vi "Flowmeter2.vi"() -> ()   [LabVIEW 2018]
uses:
  <vilib>/measure/NI_MABase.lvlib
panel:
  out "Waveform Graph 5":dynamicdata(graph)
  out "Waveform Graph 4":waveform(dbl)(graph)
  out "Waveform Graph 3":waveform(dbl)(graph)
  out "Waveform Graph 2":waveform(dbl)(graph)
  out "Waveform Graph":waveform(dbl)(graph)
  in  "Frequency2":dbl
  in  "Frequency1":dbl
  in  "Switch Modes":bool
  in  "Angle":dbl(knob) scale=90.0..30.0
  in  "Thickness of pipe":dbl
  out "Meter":dbl(knob) scale=0.0..50.0
  in  "Velocity of Fluid":dbl(slide) scale=0.0..5.0
  in  "milliseconds to wait":u32
  in  "stop":bool
  # "Electromagnetic"
  # "Ultrasonic"
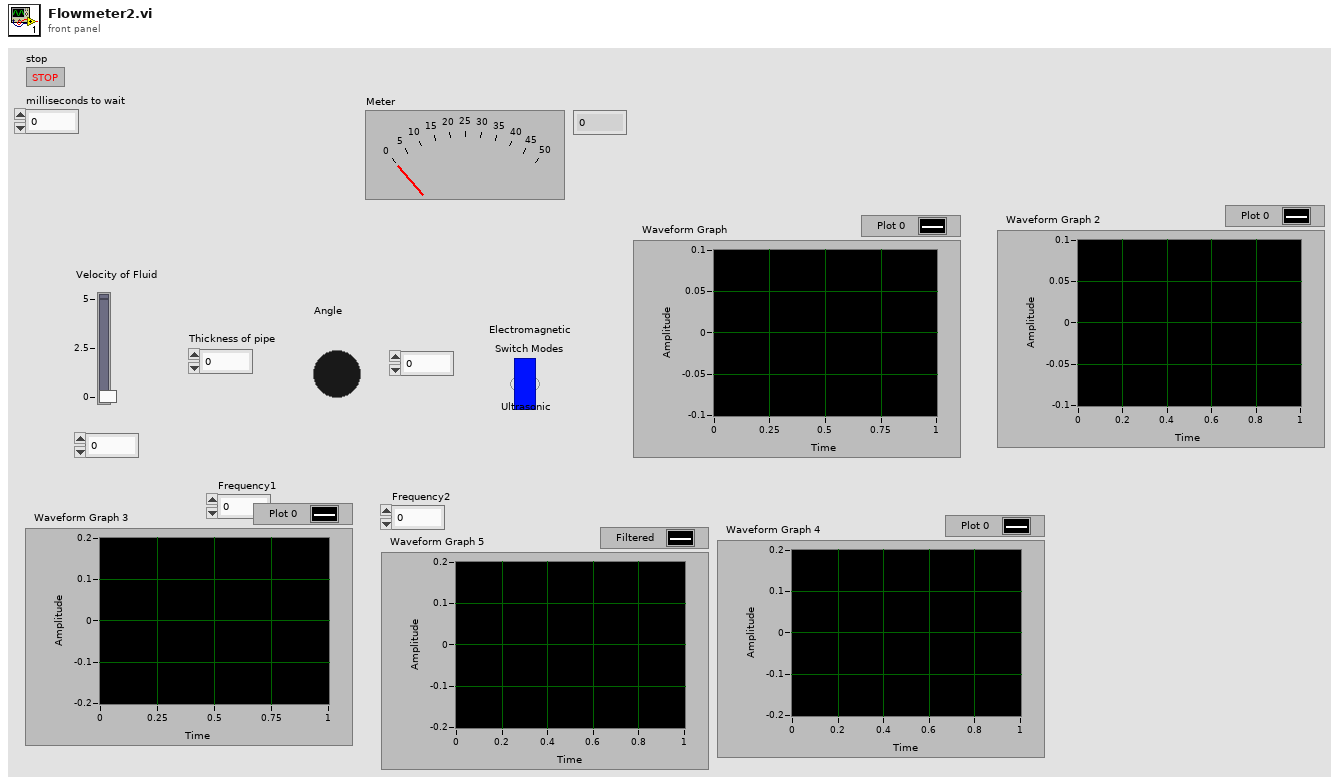
[diagram p1: front panel]
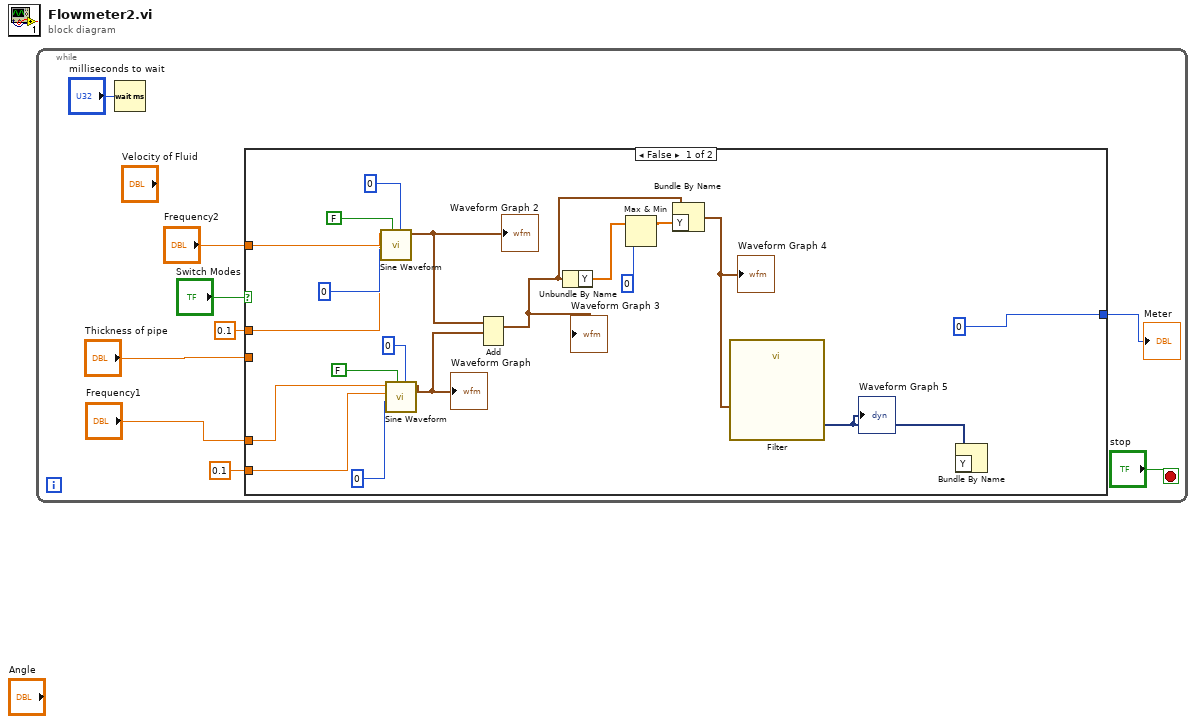
[diagram p0: block diagram]
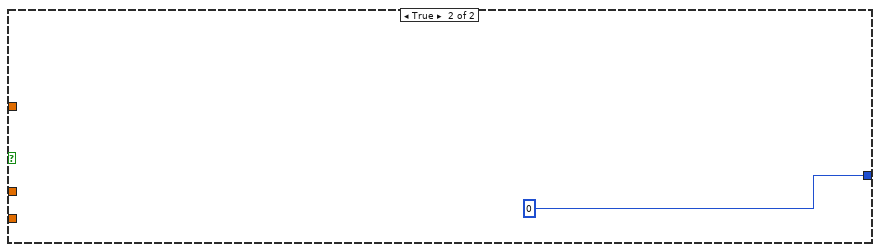
[diagram p2: hidden frame]
diagram:
  n1 = while {
    stop <- "stop" stop-if-true
    n2 = Wait (ms)(milliseconds to wait="milliseconds to wait") -> ()  [unwired: 1 out]
    n3 = case shown="False" "Switch Modes" {
      tunnel: "Thickness of pipe" -> [_ _]
      tunnel: "Frequency1" -> [w25 _]
      tunnel: "Frequency2" -> [w21 _]
      tunnel: [0 0] -> w3
      tunnel: 0.1 -> [w19 _]
      tunnel: 0.1 -> [w18 _]
      frame False {
        n4 = call <vilib>:"Sine Waveform.vi"("offset"=0, "reset signal"=FALSE, "phase"=0, "amplitude"=w18, "frequency"=w21) -> ("signal out"=w17:waveform(dbl))  [unwired: 5 in, 1 out]
        "Waveform Graph 2" <- w17
        n5 = call <vilib>:"Sine Waveform.vi"("offset"=0, "reset signal"=FALSE, "phase"=0, "amplitude"=w19, "frequency"=w25) -> ("signal out"=w16:waveform(dbl))  [unwired: 5 in, 1 out]
        "Waveform Graph" <- w16
        n6 = Add(1:w16, 2:w17) -> (0:w12:waveform(dbl))  [unwired: 1 in, 1 out]
        "Waveform Graph 3" <- w12
        n7 = Unbundle By Name(w12) -> ("Y"=w15:dbl[])
        n8 = Max & Min(x=w15, y=0) -> (max(x,y)=w13:dbl[])  [unwired: 1 out]
        n9 = Bundle By Name(cluster=w12, "Y"=w13) -> (w11:waveform(dbl))
        "Waveform Graph 4" <- w11
        n10 = call "Filter"("Signal"=w11) -> ("Filtered Signal"=w10:dynamicdata)  [unwired: 9 in, 1 out]
        "Waveform Graph 5" <- w10
        n11 = Bundle By Name(cluster=w10) -> ()  [unwired: 1 in, 1 out]
      }
      frame True {
      }
    }
    "Meter" <- w3
  }
